vi "M686_timer.vi"(1 "Reset":bool) -> (0 "Time has Elapsed":bool)   [LabVIEW 2014]
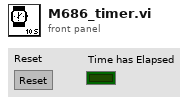
[diagram p1: front panel]
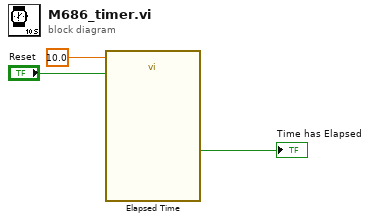
[diagram p0: block diagram]
diagram:
  n1 = call "Elapsed Time"("Time Target (s)"=10.0, "Reset"="Reset") -> ("Time has Elapsed"=→"Time has Elapsed":bool)  [unwired: 10 in, 7 out]
